vi "Read Module Page Property.vi"(8 "error in (no error)":errorcluster, 11 "Node Ptr In":T1 format="%.0x") -> (0 "error out":errorcluster, 2 "RSI Module":refnum<class "RSI Module.lvclass">, 3 "Node Ptr Out":T1 format="%.0x")   [LabVIEW 2017, in "Modules.lvlib" / "RSI Module.lvclass"]
uses:
  RSI Module.lvclass
  <vilib>/NI Veristand/Custom Device API/Custom Device Item Ref.ctl
  Debug.vi
  Class Property Strings.vi
  <vilib>/NI Veristand/Custom Device API/Get Item Property (String).vi
  <vilib>/NI Veristand/Custom Device API/Custom Device API.lvlib
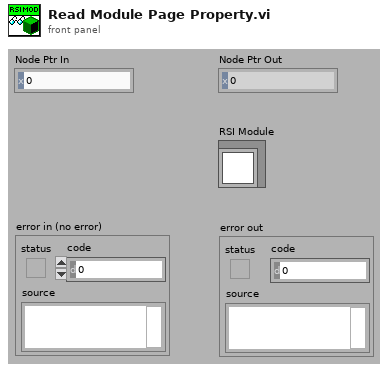
[diagram p1: front panel]
types:
  T1 = typedef "Custom Device API.lvlib/Custom Device Item Ref.ctl" = u64
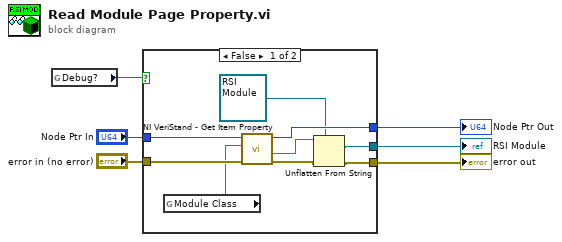
[diagram p0: block diagram]
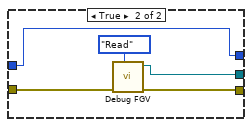
[diagram p2: hidden frame]
diagram:
  n1 = global read "Debug.vi" "Debug?"() -> (w1:bool)
  n2 = case shown="False" w1 {
    tunnel: "error in (no error)" -> [w15 w20]
    tunnel: "Node Ptr In" -> [w14 w16]
    tunnel: [w13 w16] -> w4
    tunnel: [w11 w17] -> w3
    tunnel: [w9 w18] -> w2
    frame False {
      n3 = global read "Class Property Strings.vi" "Module Class"() -> (w7:string)
      n4 = call-poly <vilib>:"NI VeriStand - Get Item Property.vi"("error in (no error)"=w15, "Property Name"=w7, "Item Ref in"=w14) -> ("error out"=w12:errorcluster, "Value"=w8:string, "Item Ref out"=w13:T1)  [unwired: 5 in, 1 out]
      n5 = Unflatten From String(type=refnum<class "RSI Module.lvclass"> refnum ("Scan Engine Custom Device.lvlib:RSI Module.lvclass"), binary string=w8, error in (no error)=w12) -> (value=w9:refnum<class "RSI Module.lvclass">, error out=w11:errorcluster)  [unwired: 2 in, 1 out]
    }
    frame True {
      n6 = call "Debug FGV.vi"("Action"=enum16{"Read", "Write"}."Read", "error in (no error)"=w20) -> ("error out"=w17:errorcluster, "RSI Module out"=w18:refnum<class "RSI Module.lvclass">)  [unwired: 8 in]
    }
  }
  "RSI Module" <- w2
  "Node Ptr Out" <- w4
  "error out" <- w3
